vi "Transparent UI.vi"() -> ()   [LabVIEW 2020]
uses:
  <vilib>/measure/NI_MABase.lvlib
panel:
  out "Waveform Graph":waveform(dbl)(graph)
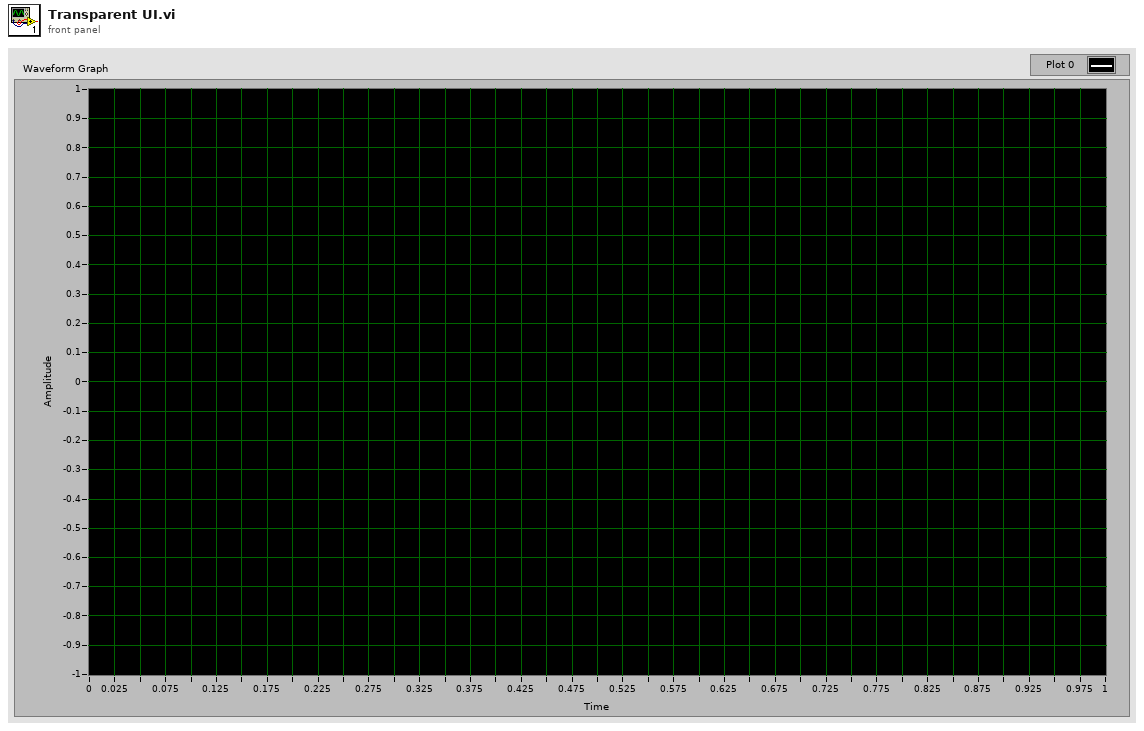
[diagram p1: front panel]
types:
  T1 = typedef "imagedata.ctl" = cluster{"image type":i32, "image depth":i32, "image":u8[], "mask":u8[], "colors":u32[], "Rectangle":cluster{"left":i16, "top":i16, "right":i16, "bottom":i16}}
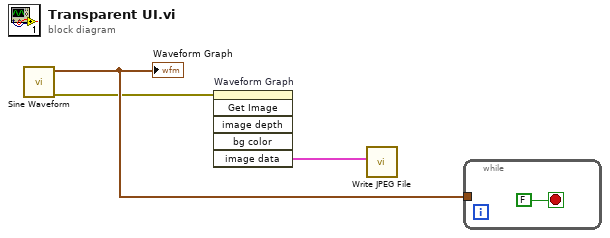
[diagram p0: block diagram]
diagram:
  n1 = call <vilib>:"Sine Waveform.vi"() -> ("error out"=w2:errorcluster, "signal out"=w3:waveform(dbl))  [unwired: 10 in]
  "Waveform Graph" <- w3
  n2 = invoke on="Waveform Graph" class="WFGraph (strict)" method="Get Image"(error in=w2) -> ("image data"=w1:T1)  [unwired: 5 in, 5 out]
  n3 = call <vilib>:"Write JPEG File.vi"("image data"=w1) -> ()  [unwired: 9 in, 2 out]
  n4 = while {
    tunnel: w3 -> [_]
    stop <- FALSE stop-if-true
  }
